vi "makeOuterMaskBox.vi"(9 "manip 1 position":T1={"width x"=498.0, "height y"=180.0, "x offset"=32.0, "y offset"=116.0}, 11 "user selected pipette tip (x,y)":i32[](array[numeric])) -> (2 "bounding box":T2, 3 "bounding rectangle":i32[](array[numeric]))   [LabVIEW 2015]
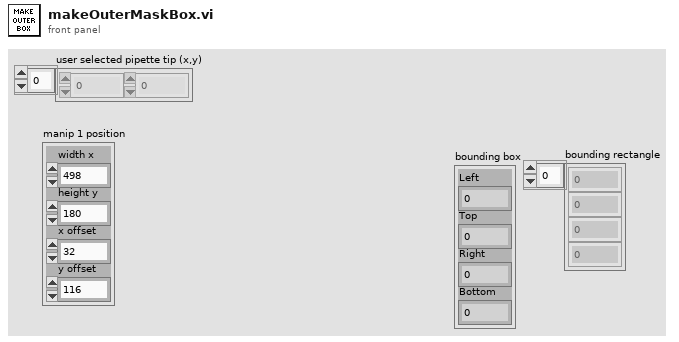
[diagram p1: front panel]
types:
  T1 = cluster{"width x":dbl, "height y":dbl, "x offset":dbl, "y offset":dbl}
  T2 = cluster{"Left":i32, "Top":i32, "Right":i32, "Bottom":i32}
  T3 = cluster{"[0]":i32, "[1]":i32, "[2]":i32, "[3]":i32}
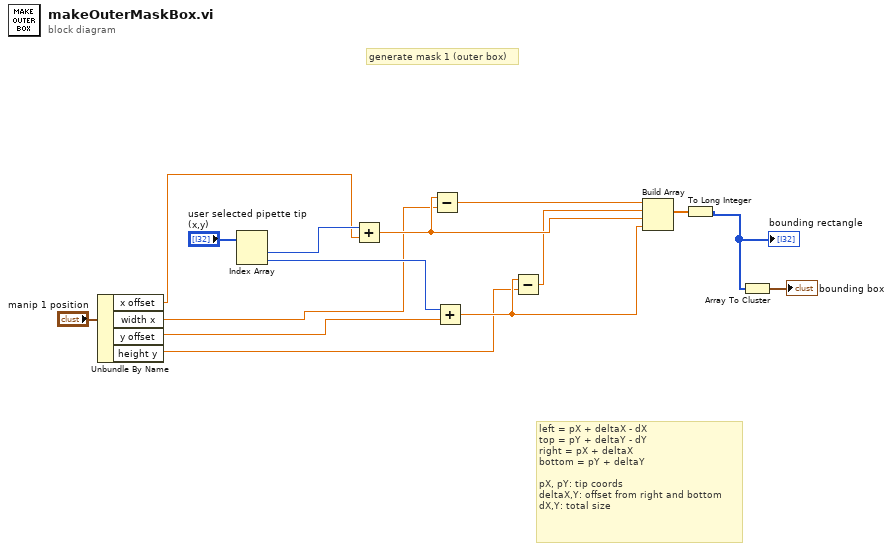
[diagram p0: block diagram]
diagram:
  # "left = pX + deltaX - dX\ntop = pY + deltaY - dY\nright = pX + deltaX\nbottom = pY + deltaY\n\npX, pY: tip coords\ndeltaX,Y: offset from right and bottom\ndX,Y: total size"
  # "generate mask 1 (outer box)"
  n1 = Unbundle By Name("manip 1 position") -> ("x offset"=w2:dbl, "width x"=w4:dbl, "y offset"=w3:dbl, "height y"=w1:dbl)
  n2 = Index Array(array="user selected pipette tip (x,y)") -> (element #1=w11:i32, element #2=w8:i32)  [unwired: 2 in]
  n3 = Add(x=w11, y=w2) -> (x+y=w10:dbl)
  n4 = Subtract(x=w10, y=w4) -> (x-y=w9:dbl)
  n5 = Add(x=w8, y=w3) -> (x+y=w7:dbl)
  n6 = Subtract(x=w7, y=w1) -> (x-y=w6:dbl)
  n7 = Build Array(w9, w6, w10, w7) -> (w15:dbl[])
  n8 = To Long Integer(number=w15) -> (32bit integer=w14:i32[])
  "bounding rectangle" <- w14
  n9 = Array To Cluster(array=w14) -> (cluster=→"bounding box":T3)
